vi "Load Configuration File.vi"(8 "error in":errorcluster, 10 "Filename":string, 11 "Camera in":refnum<class "Camera.lvclass">) -> (0 "error out":errorcluster, 2 "Supported?":bool, 3 "Camera out":refnum<class "Camera.lvclass">)   [LabVIEW 2018, in "Camera.lvlib" / "Camera.lvclass"]
uses:
  Camera.lvclass
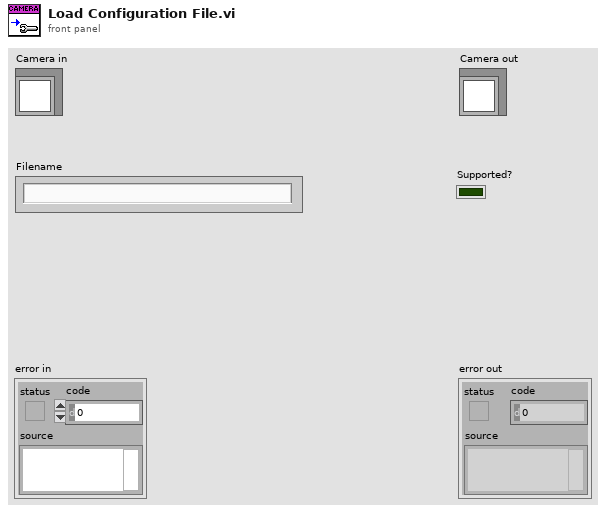
[diagram p1: front panel]
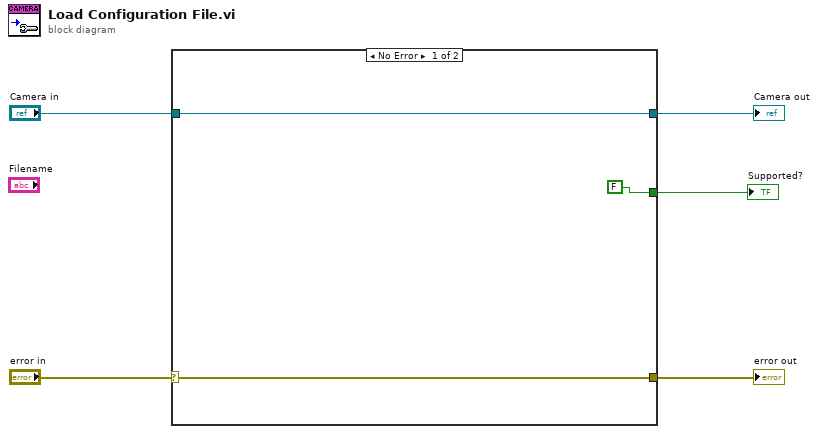
[diagram p0: block diagram]
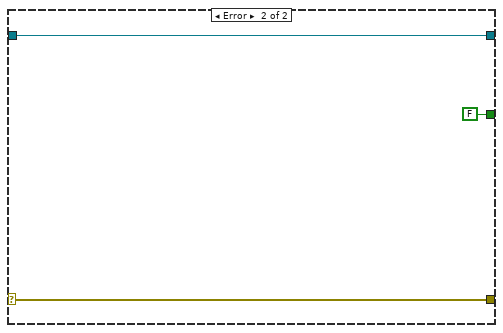
[diagram p2: hidden frame]
diagram:
  n1 = case shown="No Error" "error in" {
    selector: "error in" -> [w8 w10]
    tunnel: [w8 w10] -> w4
    tunnel: "Camera in" -> [w7 w11]
    tunnel: [w7 w11] -> w2
    tunnel: [FALSE FALSE] -> w1
    frame No Error {
    }
    frame Error {
    }
  }
  "error out" <- w4
  "Camera out" <- w2
  "Supported?" <- w1
